vi "ContourPlotAuto.vi"() -> ()   [LabVIEW 2020]
uses:
  <vilib>/Utility/file.llb/Read Delimited Spreadsheet (DBL).vi
  <vilib>/Analysis/NI_AALBase.lvlib
panel:
  in  "Tab Control":enum32{"Y cut ", "Y curve"}(tab)
  out "Y Cut":cluster{dbl[], "Intensity Graph":dbl[]}(graph)
  in  "intervals":i32=100
  out "Y Histogram":T1(graph)={"X Values"=[-0.0001131092565, -0.00011086496949999999, -0.00010862068249999998, -0.00010637639549999998, -0.00010413210849999997, -0.00010188782149999997, -9.964353449999996e-05, -9.739924749999995e-05, -9.515496049999995e-05, -9.291067349999994e-05, -9.066638649999994e-05, -8.842209949999993e-05, -8.617781249999992e-05, -8.393352549999992e-05, -8.168923849999991e-05, -7.94449514999999e-05, -7.72006644999999e-05, -7.495637749999989e-05, -7.271209049999989e-05, -7.046780349999988e-05, -6.822351649999987e-05, -6.597922949999987e-05, -6.373494249999986e-05, -6.149065549999986e-05, -5.924636849999986e-05, -5.700208149999986e-05, -5.475779449999986e-05, -5.251350749999986e-05, -5.026922049999986e-05, -4.802493349999986e-05, -4.578064649999986e-05, -4.353635949999986e-05, -4.129207249999986e-05, -3.9047785499999864e-05, -3.6803498499999865e-05, -3.4559211499999865e-05, -3.2314924499999866e-05, -3.0070637499999867e-05, -2.7826350499999868e-05, -2.5582063499999868e-05, -2.333777649999987e-05, -2.109348949999987e-05, -1.884920249999987e-05, -1.660491549999987e-05, -1.4360628499999872e-05, -1.2116341499999873e-05, -9.872054499999873e-06, -7.627767499999873e-06, -5.383480499999873e-06, -3.139193499999873e-06, -8.949064999998729e-07, 1.3493805000001272e-06, 3.5936675000001273e-06, 5.8379545000001274e-06, 8.082241500000128e-06, 1.0326528500000127e-05, 1.2570815500000126e-05, 1.4815102500000125e-05, 1.7059389500000125e-05, 1.9303676500000124e-05, 2.1547963500000123e-05, 2.3792250500000122e-05, 2.6036537500000122e-05, 2.828082450000012e-05, 3.052511150000012e-05, 3.276939850000012e-05, 3.501368550000012e-05, 3.725797250000012e-05, 3.950225950000012e-05, 4.1746546500000117e-05, 4.3990833500000116e-05, 4.6235120500000115e-05, 4.8479407500000114e-05, 5.0723694500000114e-05, 5.296798150000011e-05, 5.521226850000011e-05, 5.745655550000011e-05, 5.970084250000011e-05, 6.194512950000011e-05, 6.418941650000012e-05, 6.643370350000012e-05, 6.867799050000013e-05, 7.092227750000013e-05, 7.316656450000014e-05, 7.541085150000015e-05, 7.765513850000015e-05, 7.989942550000016e-05, 8.214371250000016e-05, 8.438799950000017e-05, 8.663228650000018e-05, 8.887657350000018e-05, 9.112086050000019e-05, 9.33651475000002e-05, 9.56094345000002e-05, 9.78537215000002e-05, 0.00010009800850000021, 0.00010234229550000022, 0.00010458658250000022, 0.00010683086950000023, 0.00010907515650000024], "Histogram: h(x)"=[64, 38, 30, 23, 26, 19, 25, 22, 21, 21, 20, 22, 21, 21, 18, 21, 21, 21, 21, 18, 20, 20, 20, 19, 21, 18, 19, 18, 20, 21, 22, 19, 19, 20, 19, 19, 19, 19, 23, 18, 18, 19, 20, 19, 18, 23, 25, 17, 20, 19, 18, 21, 21, 18, 20, 17, 20, 20, 18, 18, 19, 21, 17, 21, 19, 21, 18, 18, 18, 18, 20, 18, 19, 18, 18, 18, 18, 18, 18, 18, 19, 18, 18, 18, 18, 18, 17, 19, 15, 18, 20, 15, 19, 18, 16, 18, 19, 16, 19, 14]}
  in  "Normal T or Distribution F":bool=TRUE
  in  "book number":i32=333
  out "X Cut":cluster{dbl[], "Intensity Graph":dbl[]}(graph)
  in  "file path (dialog if empty)":path=path "\\\\ad.uillinois.edu\\engr/mrl-dvh-research/Guang Yue/data/Contour plot"
  out "Intensity Graph":dbl[][](graph)
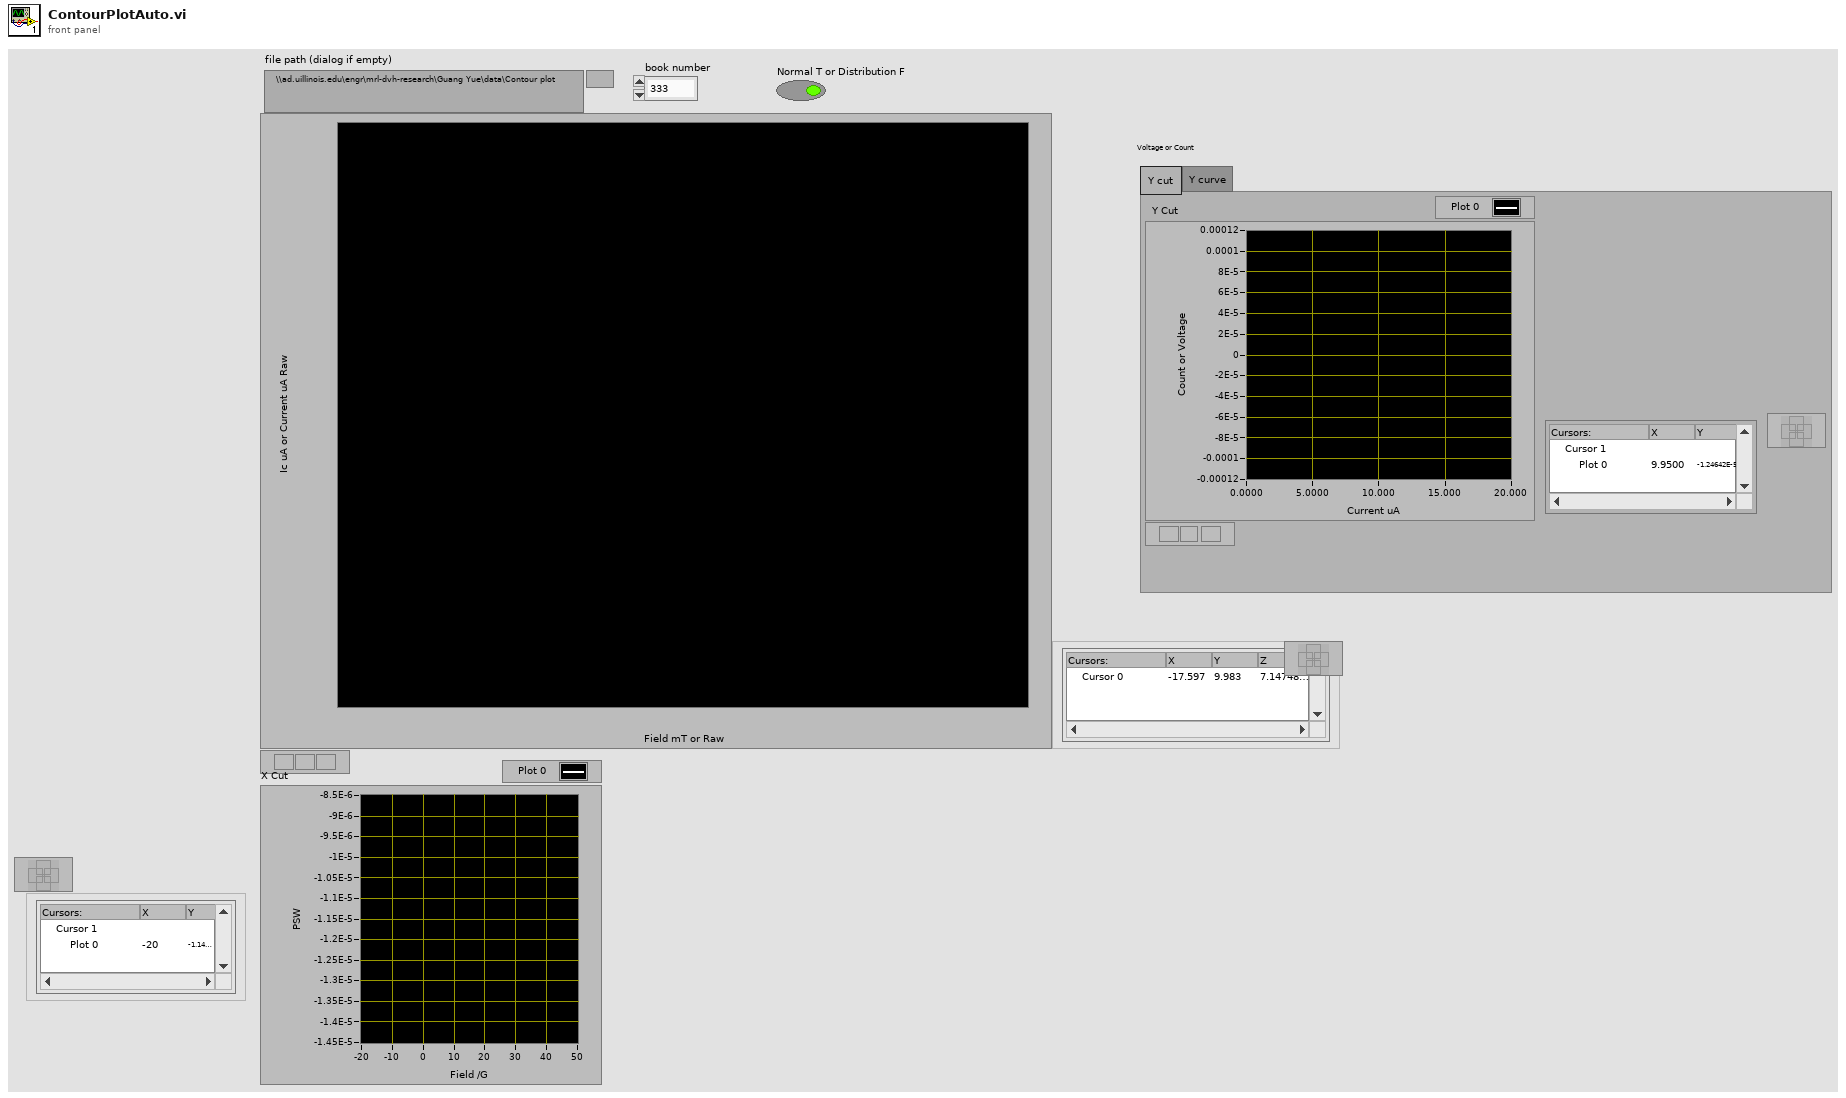
[diagram p1: front panel]
types:
  T1 = cluster{"X Values":dbl[], "Histogram: h(x)":i32[]}
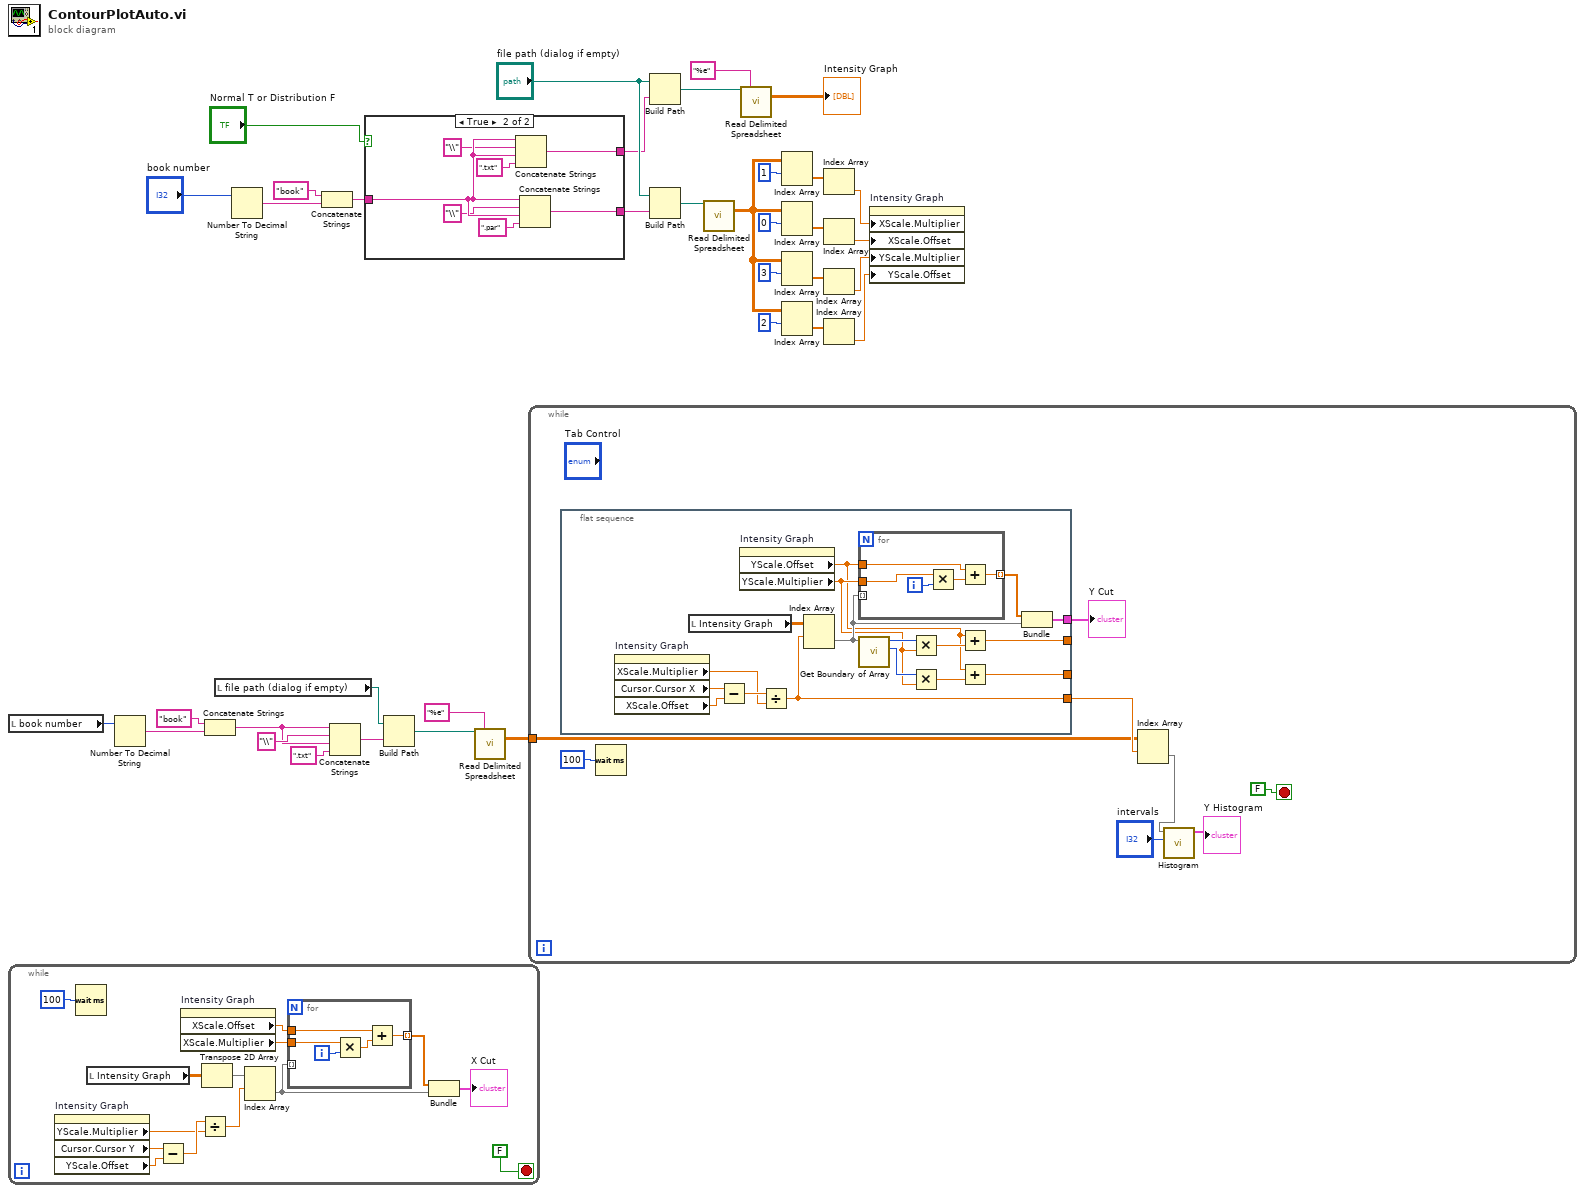
[diagram p0: block diagram]
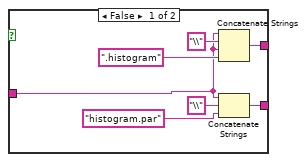
[diagram p2: hidden frame]
diagram:
  n1 = local read "book number"() -> (w34:i32)
  n2 = while {
    stop <- FALSE stop-if-true
    n3 = property on="Intensity Graph" class="IntGraph (strict)"() -> ("YScale.Multiplier"=w45:dbl, "Cursor.Cursor Y"=w44:dbl, "YScale.Offset"=w43:dbl)  [unwired: 2 in, 2 out]
    n4 = Wait (ms)(milliseconds to wait=u32 100) -> ()  [unwired: 1 out]
    n5 = local read "Intensity Graph"() -> (w40:dbl[][])
    n6 = Subtract(x=w44, y=w43) -> (x-y=w50:dbl)
    n7 = property on="Intensity Graph" class="IntGraph (strict)"() -> ("XScale.Offset"=w46:dbl, "XScale.Multiplier"=w47:dbl)  [unwired: 2 in, 2 out]
    n8 = Divide(x=w50, y=w45) -> (x/y=w49:dbl)
    n9 = Transpose 2D Array(2D array=w40) -> (transposed array=w39:dbl[][])
    n10 = Index Array(array=w39, index (row)=w49) -> (element=w41:dbl[])  [unwired: 1 in]
    n11 = for {
      tunnel: w47 -> [w54]
      tunnel: w46 -> [w52]
      tunnel: [w51] -> w48 mode=indexing
      tunnel: w41 -> [_] mode=indexing
      i -> [w55]
      n12 = Multiply(x=w54, y=w55) -> (x*y=w53:dbl)
      n13 = Add(x=w52, y=w53) -> (x+y=w51:dbl)
    }
    n14 = Bundle(w48, w41) -> (→"X Cut":cluster{dbl[], dbl[]})  [unwired: 1 in]
  }
  n15 = Number To Decimal String(number=w34) -> (decimal integer string=w36:string)  [unwired: 1 in]
  n16 = Concatenate Strings("book" ("string"), w36) -> (w31:string)
  n17 = local read "file path (dialog if empty)"() -> (w30:path)
  n18 = Number To Decimal String(number="book number") -> (decimal integer string=w19:string)  [unwired: 1 in]
  n19 = Concatenate Strings("book" ("string"), w19) -> (w21:string)
  n20 = Concatenate Strings(w31, "\\" ("string"), w31, ".txt" ("string")) -> (w29:string)
  n21 = case shown="True" "Normal T or Distribution F" {
    tunnel: [w58 w69] -> w23
    tunnel: w21 -> [w57 w67]
    tunnel: [w59 w65] -> w20
    frame False {
      n22 = Concatenate Strings(w57, "\\" ("string"), w57, ".histogram" ("string")) -> (w59:string)
      n23 = Concatenate Strings(w57, "\\" ("string"), "histogram.par" ("string")) -> (w58:string)
    }
    frame True {
      n24 = Concatenate Strings(w67, "\\" ("string"), w67, ".txt" ("string")) -> (w65:string)
      n25 = Concatenate Strings(w67, "\\" ("string"), w67, ".par" ("string")) -> (w69:string)
    }
  }
  n26 = Build Path(base path=w30, name or relative path=w29) -> (appended path=w27:path)
  n27 = call-poly <vilib>:"Read Delimited Spreadsheet.vi"("file path (dialog if empty)"=w27, "format (%.3f)"="%e") -> ("all rows"=w26:dbl[][])  [unwired: 8 in, 5 out]
  n28 = while {
    tunnel: w26 -> [w73]
    stop <- FALSE stop-if-true
    n29 = flat-sequence {
      tunnel: [w89] -> w77
      tunnel: [w81] -> _
      tunnel: [w80] -> _
      tunnel: [w79] -> w74
      frame #0 {
        n30 = property on="Intensity Graph" class="IntGraph (strict)"() -> ("XScale.Multiplier"=w92:dbl, "Cursor.Cursor X"=w91:dbl, "XScale.Offset"=w90:dbl)  [unwired: 2 in, 2 out]
        n31 = local read "Intensity Graph"() -> (w93:dbl[][])
        n32 = Subtract(x=w91, y=w90) -> (x-y=w94:dbl)
        n33 = property on="Intensity Graph" class="IntGraph (strict)"() -> ("YScale.Offset"=w82:dbl, "YScale.Multiplier"=w83:dbl)  [unwired: 2 in, 2 out]
        n34 = Divide(x=w94, y=w92) -> (x/y=w79:dbl)
        n35 = Index Array(array=w93, index (row)=w79) -> (element=w88:dbl[])  [unwired: 1 in]
        n36 = for {
          tunnel: w83 -> [w98]
          tunnel: w82 -> [w96]
          tunnel: [w95] -> w78 mode=indexing
          tunnel: w88 -> [_] mode=indexing
          i -> [w99]
          n37 = Multiply(x=w98, y=w99) -> (x*y=w97:dbl)
          n38 = Add(x=w96, y=w97) -> (x+y=w95:dbl)
        }
        n39 = call "Get Boundary of Array.vi"("Array"=w88) -> ("Up"=w84:i32, "Down"=w87:i32)  [unwired: 9 in]
        n40 = Multiply(x=w87, y=w83) -> (x*y=w86:dbl)
        n41 = Multiply(x=w84, y=w83) -> (x*y=w85:dbl)
        n42 = Add(x=w82, y=w86) -> (x+y=w81:dbl)
        n43 = Add(x=w82, y=w85) -> (x+y=w80:dbl)
        n44 = Bundle(w78, "Intensity Graph"=w88) -> (w89:cluster{dbl[], "Intensity Graph":dbl[]})  [unwired: 1 in]
      }
    }
    n45 = Wait (ms)(milliseconds to wait=u32 100) -> ()  [unwired: 1 out]
    n46 = Index Array(array=w73, index (row)=w74) -> (element=w72:dbl[])  [unwired: 1 in]
    n47 = call <vilib>:"Histogram.vi"("intervals"="intervals", "X"=w72) -> ("Histogram Graph"=→"Y Histogram":T1)  [unwired: 6 in, 3 out]
    "Y Cut" <- w77
  }
  n48 = Build Path(base path="file path (dialog if empty)", name or relative path=w20) -> (appended path=w25:path)
  n49 = Build Path(base path="file path (dialog if empty)", name or relative path=w23) -> (appended path=w24:path)
  n50 = call-poly <vilib>:"Read Delimited Spreadsheet.vi"("file path (dialog if empty)"=w24) -> ("all rows"=w15:dbl[][])  [unwired: 9 in, 5 out]
  n51 = call-poly <vilib>:"Read Delimited Spreadsheet.vi"("file path (dialog if empty)"=w25, "format (%.3f)"="%e") -> ("all rows"=→"Intensity Graph":dbl[][])  [unwired: 8 in, 5 out]
  n52 = Index Array(array=w15, index (row)=1) -> (element=w11:dbl[])  [unwired: 1 in]
  n53 = Index Array(array=w15, index (row)=0) -> (element=w12:dbl[])  [unwired: 1 in]
  n54 = Index Array(array=w15, index (row)=3) -> (element=w9:dbl[])  [unwired: 1 in]
  n55 = Index Array(array=w15, index (row)=2) -> (element=w10:dbl[])  [unwired: 1 in]
  n56 = Index Array(array=w11) -> (element=w5:dbl)  [unwired: 1 in]
  n57 = Index Array(array=w12) -> (element=w4:dbl)  [unwired: 1 in]
  n58 = Index Array(array=w9) -> (element=w3:dbl)  [unwired: 1 in]
  n59 = Index Array(array=w10) -> (element=w2:dbl)  [unwired: 1 in]
  n60 = property on="Intensity Graph" class="IntGraph (strict)"("XScale.Multiplier"=w5, "XScale.Offset"=w4, "YScale.Multiplier"=w3, "YScale.Offset"=w2) -> ()  [unwired: 2 in, 2 out]
